vi "links.vi"   [LabVIEW 2019]
uses:
  <vilib>/myRIO/Common/Instrument Driver Framework/Utilities/typedefs/Analog Scaling Constants.ctl
  <vilib>/myRIO/Common/Instrument Driver Framework/Utilities/typedefs/Analog Scaling Constants List.ctl
  <vilib>/myRIO/Common/Instrument Driver Framework/myRIO v1.0/AO/typedefs/AO Channels Enum.ctl
  <vilib>/myRIO/Common/Instrument Driver Framework/myRIO v1.0/AO/typedefs/AO Channels List.ctl
  <vilib>/myRIO/Common/Instrument Driver Framework/Utilities/typedefs/Generic FPGA Reference.ctl
  <vilib>/myRIO/Common/Instrument Driver Framework/Utilities/typedefs/myRIO v1.0 Reference.ctl
  <vilib>/myRIO/Common/Instrument Driver Framework/Utilities/typedefs/Hardware Version Enum.ctl
  <vilib>/myRIO/Common/Instrument Driver Framework/Utilities/typedefs/myRIO Generic Hardware Reference.ctl
  <vilib>/myRIO/Instrument Drivers/Onboard IO/AO/typedefs/AO Reference.ctl
  <vilib>/myRIO/Instrument Drivers/Onboard IO/AO/AO.lvlib
  <vilib>/myRIO/Instrument Drivers/Onboard IO/AO/vis/Write.vi
  <vilib>/userDefined/High Color/nirio_resource_hc.ctl
  <vilib>/myRIO/Common/Instrument Driver Framework/myRIO v1.0/AO/vis/myRIO v1.1 Open AO.vi
  <vilib>/myRIO/Instrument Drivers/Onboard IO/AO/vis/myRIO AO Open.xnode
  <vilib>/myRIO/Common/Instrument Driver Framework/Utilities/vis/Is FPGA Ref Available.vi
  <vilib>/myRIO/Express VI/Onboard IO/AO/AO Express VI.xnode
  interface.vi
  <vilib>/myRIO/Common/Instrument Driver Framework/myRIO v1.0/DIO/typedefs/DIO Channels Enum.ctl
  <vilib>/myRIO/Common/Instrument Driver Framework/myRIO v1.0/DIO/typedefs/DIO Channels List.ctl
  <vilib>/myRIO/Instrument Drivers/Onboard IO/DIO/typedefs/DIO Reference.ctl
  <vilib>/myRIO/Instrument Drivers/Onboard IO/DIO/DIO.lvlib
  <vilib>/myRIO/Instrument Drivers/Onboard IO/DIO/vis/Read.vi
  <vilib>/myRIO/Instrument Drivers/Onboard IO/DIO/vis/myRIO DIO Open.xnode
  <vilib>/myRIO/Express VI/Onboard IO/DI/DI Express VI.xnode
  <vilib>/myRIO/Common/Instrument Driver Framework/myRIO v1.0/DIO/vis/myRIO v1.1 Open DIO.vi
types:
  T1 = typedef "AO.lvlib/AO Reference.ctl" = cluster{"myRIO Reference":T2, "AO Channel List":T6, "AO Scaling Constant List":T8}
  T2 = typedef "myRIO Generic Hardware Reference.ctl" = cluster{"myRIO Model":T3, "myRIO Hardware Reference":T4}
  T3 = typedef "Hardware Version Enum.ctl" = enum16{"Unknown", "myRIO-1900", "myRIO-1950", "roboRIO", "NI ELVIS RIO CM", "ELVIS III"}
  T4 = typedef "myRIO v1.0 Reference.ctl" = cluster{"Generic FPGA Reference":T5, "Allow multiple opens":bool}
  T5 = typedef "Generic FPGA Reference.ctl" = refnum<k20>
  T6 = typedef "AO Channels List.ctl" = T7[]
  T7 = typedef "AO Channels Enum.ctl" = enum16{"Not Connected", "AudioOut/Left", "AudioOut/Right", "C/AO0", "C/AO1", "A/AO0", "A/AO1", "B/AO0", "B/AO1"}
  T8 = typedef "Analog Scaling Constants List.ctl" = T9[]
  T9 = typedef "Analog Scaling Constants.ctl" = cluster{"LSB Weight (Volts)":dbl, "Offset (Volts)":dbl, "Signed?":bool}
  T10 = typedef "nirio_resource_hc.ctl" = tag
  T11 = typedef "DIO.lvlib/DIO Reference.ctl" = cluster{"myRIO Reference":T2, "DIO Channels List":T12}
  T12 = typedef "DIO Channels List.ctl" = T13[]
  T13 = typedef "DIO Channels Enum.ctl" = enum16{"Not Connected", "C/DIO0", "C/DIO1", "C/DIO2", "C/DIO3", "C/DIO4", "C/DIO5", "C/DIO6", "C/DIO7", "A/DIO0", "A/DIO1", "A/DIO2", "A/DIO3", "A/DIO4", "A/DIO5", "A/DIO6", "A/DIO7", "A/DIO8", "A/DIO9", "A/DIO10", "A/DIO11", "A/DIO12", "A/DIO13", "A/DIO14", "A/DIO15", "A/DIO16", "A/DIO17", "A/DIO18", "A/DIO19", "B/DIO0", "B/DIO1", "B/DIO2", "B/DIO3", "B/DIO4", "B/DIO5", "B/DIO6", "B/DIO7", "B/DIO8", "B/DIO9", "B/DIO10", "B/DIO11", "B/DIO12", "B/DIO13", "B/DIO14", "B/DIO15", "B/DIO16", "B/DIO17", "B/DIO18", "B/DIO19", "LED0", "LED1", "LED2", "LED3", "Button0", "DIO/DIO0", "DIO/DIO1", "DIO/DIO2", "DIO/DIO3", "DIO/DIO4", "DIO/DIO5", "DIO/DIO6", "DIO/DIO7", "DIO/DIO8", "DIO/DIO9", "SPI/CS0", "SPI/CS1", "SPI/CS2", "SPI/CS3", "LED RADIO (Green)", "LED RADIO (Red)", "LED COMM (Green)", "LED COMM (Red)", "LED MODE (Green)", "LED MODE (Red)"}
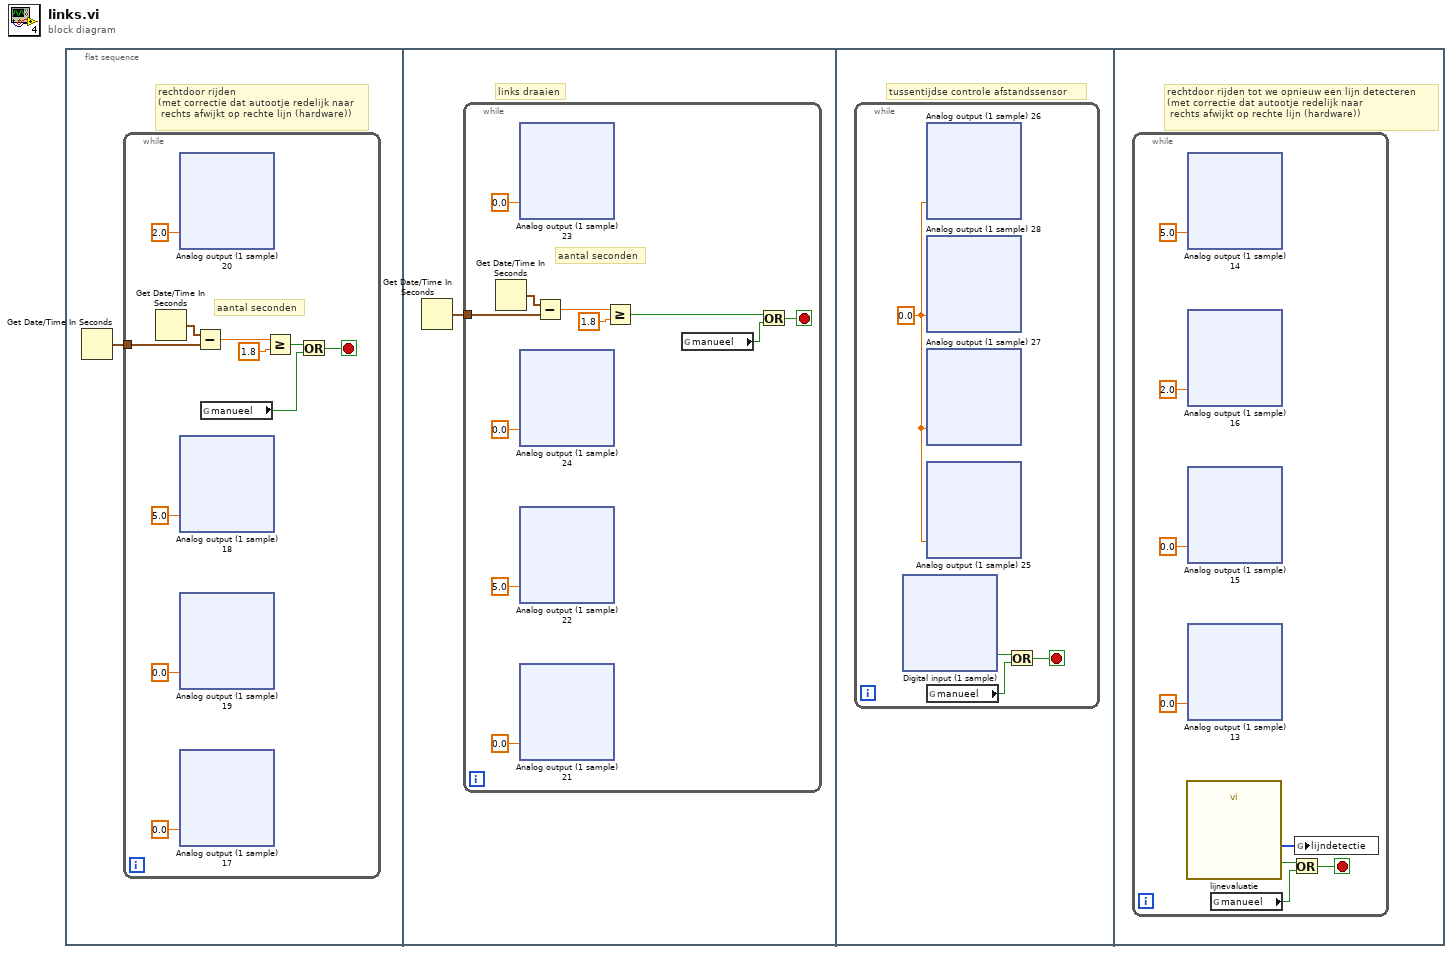
[diagram p0: block diagram]
diagram:
  n1 = flat-sequence {
    frame #0 {
      # "rechtdoor rijden\n(met correctie dat autootje redelijk naar\n rechts afwijkt op rechte lijn (hardware))"
      n2 = Get Date/Time In Seconds() -> (seconds since 1Jan1904=w1:timestamp)
      n3 = while {
        tunnel: w1 -> [w6]
        stop <- w4 stop-if-true
        # "aantal seconden"
        n4 = Get Date/Time In Seconds() -> (seconds since 1Jan1904=w7:timestamp)
        n5 = xnode "Analog output (1 sample) 20"("A/AO0 (Pin 2)"=2.0) -> ()  [unwired: 1 in, 1 out]
        n6 = xnode "Analog output (1 sample) 18"("B/AO0 (Pin 2)"=5.0) -> ()  [unwired: 1 in, 1 out]
        n7 = xnode "Analog output (1 sample) 19"("A/AO1 (Pin 4)"=0.0) -> ()  [unwired: 1 in, 1 out]
        n8 = xnode "Analog output (1 sample) 17"("B/AO1 (Pin 4)"=0.0) -> ()  [unwired: 1 in, 1 out]
        n9 = Subtract(x=w7, y=w6) -> (x-y=w8:dbl)
        n10 = global read "interface.vi" "manueel"() -> (w5:bool)
        n11 = Greater Or Equal?(x=w8, y=1.8) -> (x >= y?=w3:bool)
        n12 = Or(x=w3, y=w5) -> (x .or. y?=w4:bool)
      }
    }
    frame #1 {
      # "links draaien"
      n13 = Get Date/Time In Seconds() -> (seconds since 1Jan1904=w161:timestamp)
      n14 = while {
        tunnel: w161 -> [w166]
        stop <- w163 stop-if-true
        # "aantal seconden"
        n15 = Get Date/Time In Seconds() -> (seconds since 1Jan1904=w167:timestamp)
        n16 = xnode "Analog output (1 sample) 23"("A/AO1 (Pin 4)"=0.0) -> ()  [unwired: 1 in, 1 out]
        n17 = xnode "Analog output (1 sample) 24"("A/AO0 (Pin 2)"=0.0) -> ()  [unwired: 1 in, 1 out]
        n18 = xnode "Analog output (1 sample) 22"("B/AO0 (Pin 2)"=5.0) -> ()  [unwired: 1 in, 1 out]
        n19 = xnode "Analog output (1 sample) 21"("B/AO1 (Pin 4)"=0.0) -> ()  [unwired: 1 in, 1 out]
        n20 = Subtract(x=w167, y=w166) -> (x-y=w168:dbl)
        n21 = Greater Or Equal?(x=w168, y=1.8) -> (x >= y?=w164:bool)
        n22 = global read "interface.vi" "manueel"() -> (w165:bool)
        n23 = Or(x=w164, y=w165) -> (x .or. y?=w163:bool)
      }
    }
    frame #2 {
      # "tussentijdse controle afstandssensor"
      n24 = while {
        stop <- w322 stop-if-true
        w324 = 0.0
        n25 = xnode "Digital input (1 sample)"() -> ("A/DIO1 (Pin 13)"=w323:bool)  [unwired: 1 in, 1 out]
        n26 = xnode "Analog output (1 sample) 26"("A/AO1 (Pin 4)"=w324) -> ()  [unwired: 1 in, 1 out]
        n27 = xnode "Analog output (1 sample) 28"("B/AO0 (Pin 2)"=w324) -> ()  [unwired: 1 in, 1 out]
        n28 = xnode "Analog output (1 sample) 27"("A/AO0 (Pin 2)"=w324) -> ()  [unwired: 1 in, 1 out]
        n29 = xnode "Analog output (1 sample) 25"("B/AO1 (Pin 4)"=w324) -> ()  [unwired: 1 in, 1 out]
        n30 = global read "interface.vi" "manueel"() -> (w321:bool)
        n31 = Or(x=w323, y=w321) -> (x .or. y?=w322:bool)
      }
    }
    frame #3 {
      # "rechtdoor rijden tot we opnieuw een lijn detecteren\n(met correctie dat autootje redelijk naar\n rechts afwijkt op rechte lijn (hardware))"
      n32 = while {
        stop <- w511 stop-if-true
        n33 = call "lijnevaluatie.vi"() -> ("digitaal lijn 0-1"=w510:i32[], "lijn gedecteerd"=w509:bool)  [unwired: 8 in, 2 out]
        n34 = xnode "Analog output (1 sample) 14"("B/AO0 (Pin 2)"=5.0) -> ()  [unwired: 1 in, 1 out]
        n35 = xnode "Analog output (1 sample) 16"("A/AO0 (Pin 2)"=2.0) -> ()  [unwired: 1 in, 1 out]
        n36 = xnode "Analog output (1 sample) 15"("A/AO1 (Pin 4)"=0.0) -> ()  [unwired: 1 in, 1 out]
        n37 = xnode "Analog output (1 sample) 13"("B/AO1 (Pin 4)"=0.0) -> ()  [unwired: 1 in, 1 out]
        n38 = global read "interface.vi" "manueel"() -> (w512:bool)
        n39 = Or(x=w509, y=w512) -> (x .or. y?=w511:bool)
        n40 = global write "interface.vi" "lijndetectie"(w510) -> ()
      }
    }
  }
